vi "Set Amplitude.vi"(7 "Channel Name (1)":u8(ring)=1 items=["1"=1, "2"=2, "3"=3, "4"=4], 8 "error in (no error)":errorcluster, 10 "Amplitude V":dbl=5.0, 11 "VISA resource name":refnum<visa-resource-name>="GPIB0::1::INSTR") -> (0 "error out":errorcluster)   [LabVIEW 2021]
uses:
  <instrlib>/Tektronix AWG 5000 7000 Series/Tektronix AWG 5000 7000 Series.lvlib
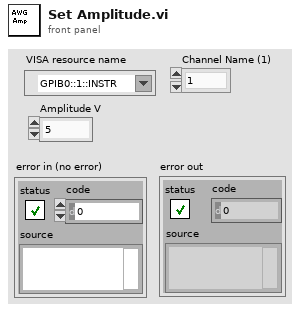
[diagram p1: front panel]
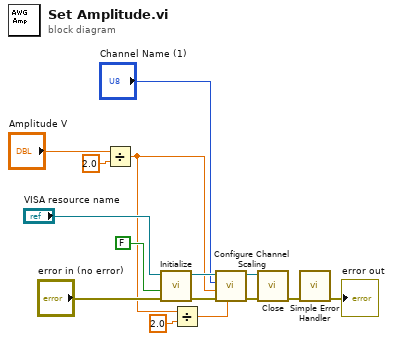
[diagram p0: block diagram]
diagram:
  n1 = Divide(x="Amplitude V", y=2.0) -> (x/y=w3:dbl)
  n2 = call <instrlib>:"Initialize.vi"("error in (no error)"="error in (no error)", "Reset (False)"=FALSE ("Reset? (F: No)"), "VISA resource name"="VISA resource name") -> ("error out"=w10:errorcluster, "VISA resource name out"=w9:refnum<visa-resource-name>)  [unwired: 7 in]
  n3 = Divide(x=w3, y=2.0) -> (x/y=w1:dbl)
  n4 = call <instrlib>:"Configure Channel Scaling.vi"("Offset (0 V)"=w1, "error in (no error)"=w10, "Amplitude (0.5 Vpp)"=w3, "Channel Name (1)"="Channel Name (1)", "VISA resource name"=w9) -> ("error out"=w7:errorcluster, "VISA resource name out"=w8:refnum<visa-resource-name>)  [unwired: 5 in]
  n5 = call <instrlib>:"Close.vi"("error in (no error)"=w7, "VISA resource name"=w8) -> ("error out"=w12:errorcluster)  [unwired: 9 in]
  n6 = call <vilib>:"Simple Error Handler.vi"("error in (no error)"=w12) -> ("error out"=→"error out":errorcluster)  [unwired: 4 in, 4 out]
